vi "(SubVI)Launcher_Edition Check from File.vi"(7 "Function":T2, 10 "SN":string, 11 "Edition in":T1) -> (3 "Edition out":T1)   [LabVIEW 2020]
uses:
  Controls/(Ctrl)Launcher_Edition Check form File_Function.ctl
  Controls/(Ctrl)Launcher_RedNoah3 Edition.ctl
  <vilib>/Utility/config.llb/Read Key (String).vi
  <vilib>/Utility/config.llb/Write Key (String).vi
  <vilib>/Utility/config.llb/NI_LVConfig.lvlib
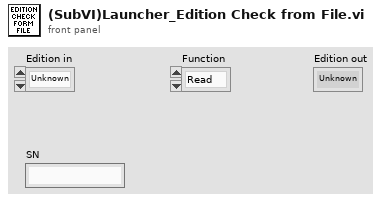
[diagram p1: front panel]
types:
  T1 = typedef "(Ctrl)Launcher_RedNoah3 Edition.ctl" = enum16{"Unknown", "Single Board", "Sensor Package"}
  T2 = typedef "(Ctrl)Launcher_Edition Check form File_Function.ctl" = enum16{"Read", "Write"}
  T3 = typedef "NI_LVConfig.lvlib/Config Data RefNum.ctl" = refnum<k1>
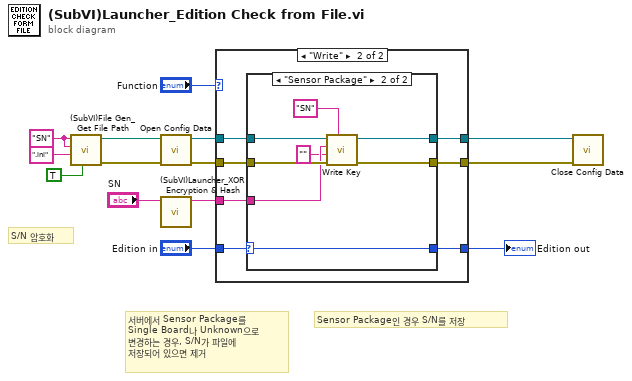
[diagram p0: block diagram]
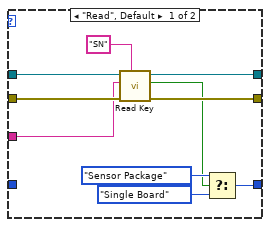
[diagram p2: hidden frame]
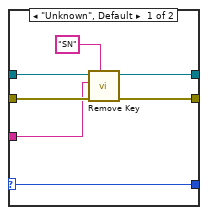
[diagram p3: hidden frame]
diagram:
  w11 = "SN" ("Folder Name")
  # "S/N 암호화"
  # "Sensor Package인 경우 S/N를 저장"
  # "서버에서 Sensor Package를\nSingle Board나 Unknown으로\n변경하는 경우, S/N가 파일에\n저장되어 있으면 제거"
  n1 = call "(SubVI)File Gen_Get File Path.vi"("Common?"=TRUE, "File Extension (.txt)"=".ini", "File Name"=w11, "Folder Name"=w11) -> ("error out"=w14:errorcluster, "Path"=w13:path)  [unwired: 5 in, 1 out]
  n2 = call <vilib>:"Open Config Data.vi"("error in (no error)"=w14, "configuration file path"=w13) -> ("error out"=w7:errorcluster, "refnum"=w8:T3)  [unwired: 7 in, 1 out]
  n3 = call "(SubVI)Launcher_XOR Encryption & Hash.vi"("Plain Text"="SN") -> ("Digest"=w6:string)  [unwired: 8 in, 2 out]
  n4 = case shown="\"Write\"" "Function" {
    tunnel: w8 -> [w20 w29]
    tunnel: w7 -> [w24 w31]
    tunnel: w6 -> [w21 w27]
    tunnel: [w19 w28] -> w4
    tunnel: [w23 w30] -> w3
    tunnel: [w16 w25] -> w2
    tunnel: "Edition in" -> [_ w26]
    frame "Read", Default {
      n5 = call-poly <vilib>:"Read Key.vi"("section"="SN", "error in (no error)"=w24, "key"=w21, "refnum"=w20) -> ("error out"=w23:errorcluster, "found?"=w17:bool, "refnum out"=w19:T3)  [unwired: 4 in, 1 out]
      n6 = Select(t=(Ctrl)Launcher_RedNoah3_Edition."Sensor Package" ("Edition in"), s=w17, f=(Ctrl)Launcher_RedNoah3_Edition."Single Board") -> (s? t:f=w16:T1)
    }
    frame "Write" {
      n7 = case shown="\"Sensor Package\"" w26 {
        selector: w26 -> [w38 w39]
        tunnel: w31 -> [w37 w46]
        tunnel: [w36 w45] -> w30
        tunnel: w29 -> [w35 w44]
        tunnel: [w34 w43] -> w28
        tunnel: w27 -> [w32 w41]
        tunnel: [w38 w39] -> w25
        frame "Unknown", Default {
          n8 = call <vilib>:"Remove Key.vi"("section"="SN", "error in (no error)"=w37, "key"=w32, "refnum"=w35) -> ("error out"=w36:errorcluster, "refnum out"=w34:T3)  [unwired: 5 in, 1 out]
        }
        frame "Sensor Package" {
          n9 = call-poly <vilib>:"Write Key.vi"("section"="SN", "error in (no error)"=w46, "value"="", "key"=w41, "refnum"=w44) -> ("error out"=w45:errorcluster, "refnum out"=w43:T3)  [unwired: 4 in, 1 out]
        }
      }
    }
  }
  "Edition out" <- w2
  n10 = call <vilib>:"Close Config Data.vi"("error in (no error)"=w3, "refnum"=w4) -> ()  [unwired: 8 in, 2 out]
